vi "Create Channels.vi"(8 "error in (no error)":errorcluster, 10 "RSI Module in":refnum<class "9217.lvclass">, 11 "Parent Ref in":T1 format="%.0x") -> (0 "error out":errorcluster, 2 "RSI Module out":refnum<class "9217.lvclass">, 3 "Parent Ref out":T1 format="%.0x")   [LabVIEW 2020, in "Modules.lvlib" / "9217.lvclass"]
uses:
  9217.lvclass
  C:/Users/nitest/Desktop/Git 2020/niveristand-scan-engine-module-libraries/Source/RSI Module/RSI Module.lvclass
  <vilib>/NI VeriStand/Custom Device API/Custom Device Item Ref.ctl
  <vilib>/NI VeriStand/Custom Device API/Custom Device Channel Type.ctl
  <vilib>/NI VeriStand/Custom Device API/Custom Device Channel.ctl
  RSI Module/Class Property Strings.vi
  RSI Module/Channel GUIDs.vi
  <vilib>/NI VeriStand/Custom Device API/Custom Device API.lvlib
  RSI Module/RSI Module.lvclass
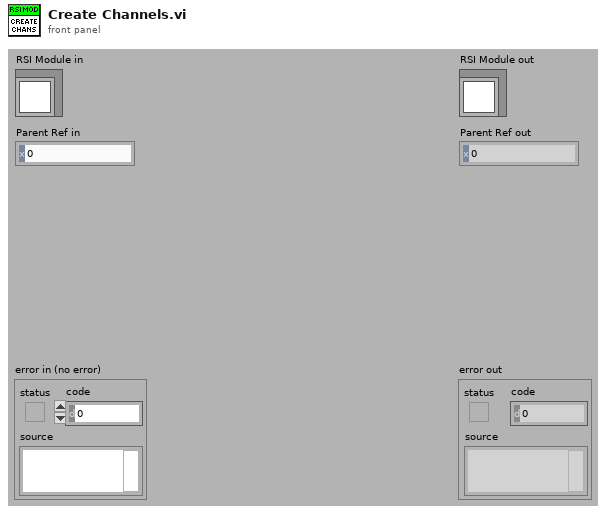
[diagram p1: front panel]
types:
  T1 = typedef "Custom Device API.lvlib/Custom Device Item Ref.ctl" = u64
  T2 = typedef "Custom Device API.lvlib/Custom Device Channel.ctl" = cluster{"Type":T3, "Units":string, "Default Value":dbl, "Faultable":bool, "Scalable":bool}
  T3 = typedef "Custom Device API.lvlib/Custom Device Channel Type.ctl" = enum16{"Input", "Output"}
  T4 = typedef "Modules.lvlib/RSI Module.lvclass/Channels.ctl" = cluster{"# Input Channels":i32, "# Output Channels":i32, "Channel Type":T5, "Units":string}
  T5 = typedef "Modules.lvlib/RSI Module.lvclass/Channel Type.ctl" = enum16{"Analog", "Digital"}
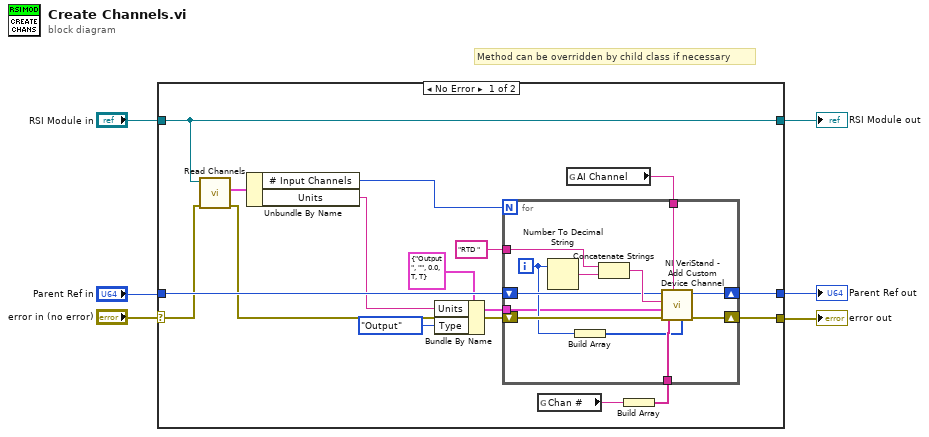
[diagram p0: block diagram]
diagram:
  # "Method can be overridden by child class if necessary"
  n1 = case shown="No Error" "error in (no error)" {
    selector: "error in (no error)" -> [w15 w37]
    tunnel: [w19 w37] -> w5
    tunnel: [w10 w36] -> w3
    tunnel: "RSI Module in" -> [w10 w36]
    tunnel: "Parent Ref in" -> [w22 w35]
    tunnel: [w18 w35] -> w1
    frame No Error {
      n2 = call "Read Channels.vi"("error in (no error)"=w15, "RSI Module in"=w10) -> ("error out"=w14:errorcluster, "Channels"=w16:T4)  [unwired: 7 in, 1 out]
      n3 = Unbundle By Name(w16) -> ("# Input Channels"=w9:i32, "Units"=w17:string)
      n4 = Bundle By Name(cluster=T2 {"Type"=enum."Output", "Units"="", "Default Value"=0.0, "Faultable"=TRUE, "Scalable"=TRUE} ("Channel"), "Units"=w17, "Type"=Custom_Device_Channel_Type."Output") -> (w11:T2)
      n5 = global read "Class Property Strings.vi" "Chan #"() -> (w21:string)
      n6 = global read "Channel GUIDs.vi" "AI Channel"() -> (w8:string)
      n7 = Build Array(w21) -> (w20:string[])
      n8 = for {
        N: w9 -> [_]
        tunnel: "RTD " ("Channel Name") -> [w32]
        tunnel: w11 -> [w23]
        tunnel: w8 -> [w24]
        tunnel: w20 -> [w29]
        shift-right: [w26] -> w19
        shift-left: w14 -> [w33]
        shift-right: [w25] -> w18
        shift-left: w22 -> [w30]
        i -> [w28]
        n9 = Number To Decimal String(number=w28) -> (decimal integer string=w34:string)  [unwired: 1 in]
        n10 = Build Array(w28) -> (w27:i32[])
        n11 = Concatenate Strings(w32, w34) -> (w31:string)
        n12 = call <vilib>:"NI VeriStand - Add Custom Device Channel.vi"("Property Values"=w27, "Property names"=w29, "GUID (Default Channel)"=w24, "error in (no error)"=w33, "Channel"=w23, "Channel Name"=w31, "Parent Ref in"=w30) -> ("error out"=w26:errorcluster, "Parent Ref out"=w25:T1)  [unwired: 1 in, 2 out]
      }
    }
    frame Error {
    }
  }
  "error out" <- w5
  "RSI Module out" <- w3
  "Parent Ref out" <- w1
